vi "RgbaToU64vi.vi"(11 "Rgba":T1) -> (3 "U64":u64)   [LabVIEW 2024, in "OpenLvVision_Image.lvlib" / "DataAccess.lvlib"]
doc: "Convert an color cluster into an number"
uses:
  DataAccess.lvlib
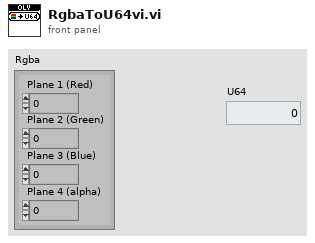
[diagram p1: front panel]
types:
  T1 = typedef "Color (U64)" = cluster{"Plane 3 (Blue)":u16, "Plane 2 (Green)":u16, "Plane 1 (Red)":u16, "Plane 4 (alpha)":u16}
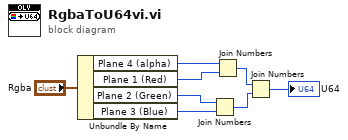
[diagram p0: block diagram]
diagram:
  n1 = Unbundle By Name("Rgba") -> ("Plane 4 (alpha)"=w6:u16, "Plane 1 (Red)"=w5:u16, "Plane 2 (Green)"=w4:u16, "Plane 3 (Blue)"=w3:u16)
  n2 = Join Numbers(hi=w4, lo=w3) -> ((hi.lo)=w7:u32)
  n3 = Join Numbers(hi=w6, lo=w5) -> ((hi.lo)=w8:u32)
  n4 = Join Numbers(hi=w8, lo=w7) -> ((hi.lo)=→"U64":u64)
